vi "Delete Files by Pattern.vi"(8 "error in (no error)":errorcluster, 10 "pattern":string="cal_*.csv", 11 "Path":path) -> (0 "error out":errorcluster, 2 "Files Deleted":path[](array[path]))   [LabVIEW 2025, in "File System.lvlib"]
uses:
  File System.lvlib
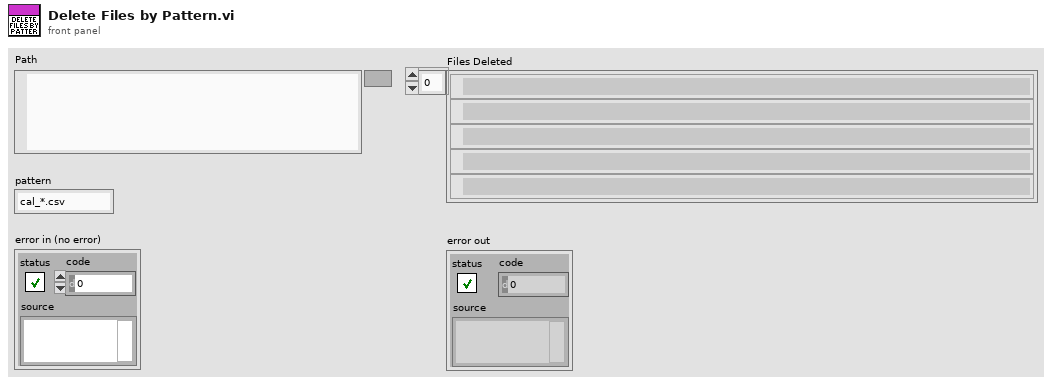
[diagram p1: front panel]
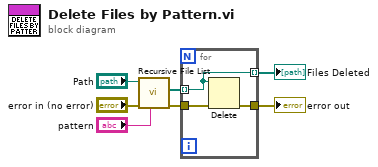
[diagram p0: block diagram]
diagram:
  n1 = call <vilib>:"Recursive File List.vi"("pattern"="pattern", "error in (no error)"="error in (no error)", "Folder Path"="Path") -> ("error out"=w4:errorcluster, "All Files in Dir"=w3:path[])  [unwired: 4 in, 3 out]
  n2 = for {
    tunnel: w3 -> [w8] mode=indexing
    tunnel: w4 -> [w10]
    tunnel: [w9] -> w2
    tunnel: [w8] -> w1 mode=indexing
    n3 = Delete(path (use dialog)=w8, error in=w10) -> (error out=w9:errorcluster)  [unwired: 3 in, 2 out]
  }
  "error out" <- w2
  "Files Deleted" <- w1
